vi "Disconnect.vi"(8 "error in":errorcluster, 11 "69X_79X in":refnum<class "6972A.lvclass">) -> (0 "error out":errorcluster, 3 "69X_79X out":refnum<class "6972A.lvclass">)   [LabVIEW 2019, in "6972A.lvlib" / "6972A.lvclass"]
uses:
  Library/6972A.lvclass
  Library/6972A.lvclass/6972A.ctl
  <instrlib>/Agilent N6900 N7900 Series/Agilent N6900 N7900 Series.lvlib
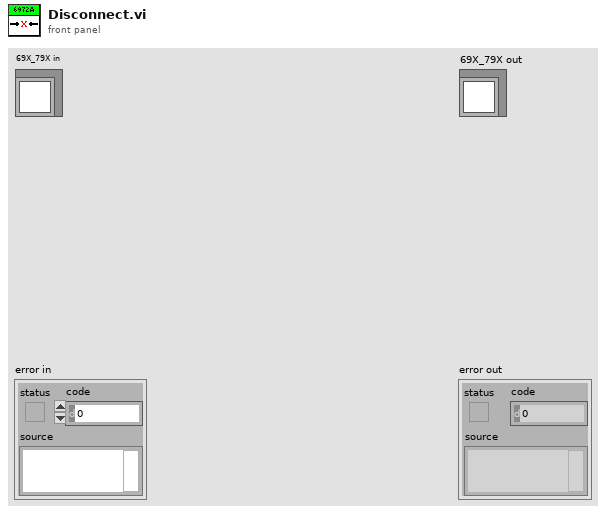
[diagram p1: front panel]
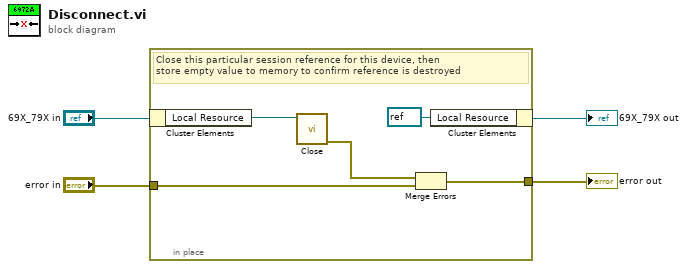
[diagram p0: block diagram]
diagram:
  n1 = in-place {
    in-place-border: "error in" -> [w9]
    in-place-border: [w8] -> w2
    # "Close this particular session reference for this device, then\nstore empty value to memory to confirm reference is destroyed"
    n2 = in-place-cluster #1("69X_79X in") -> ("Local Resource"=w6:refnum<visa-resource-name>)
    n3 = call <instrlib>:"Close.vi"("VISA resource name"=w6) -> ("error out"=w5:errorcluster)  [unwired: 10 in]
    n4 = Merge Errors(w5, w9) -> (w8:errorcluster)
    n5 = in-place-cluster #1("Local Resource"=refnum<visa-resource-name> refnum) -> (→"69X_79X out":refnum<class "6972A.lvclass">)
  }
  "error out" <- w2
